vi "as_saveStimList.vi"(4 "error in (no error)":errorcluster, 6 "Stimulus List":dbl[][](array[numeric]), 7 "Path In":path) -> (0 "error out":errorcluster, 3 "Path":path)   [LabVIEW 2009]
uses:
  <vilib>/Utility/file.llb/Write To Spreadsheet File (DBL).vi
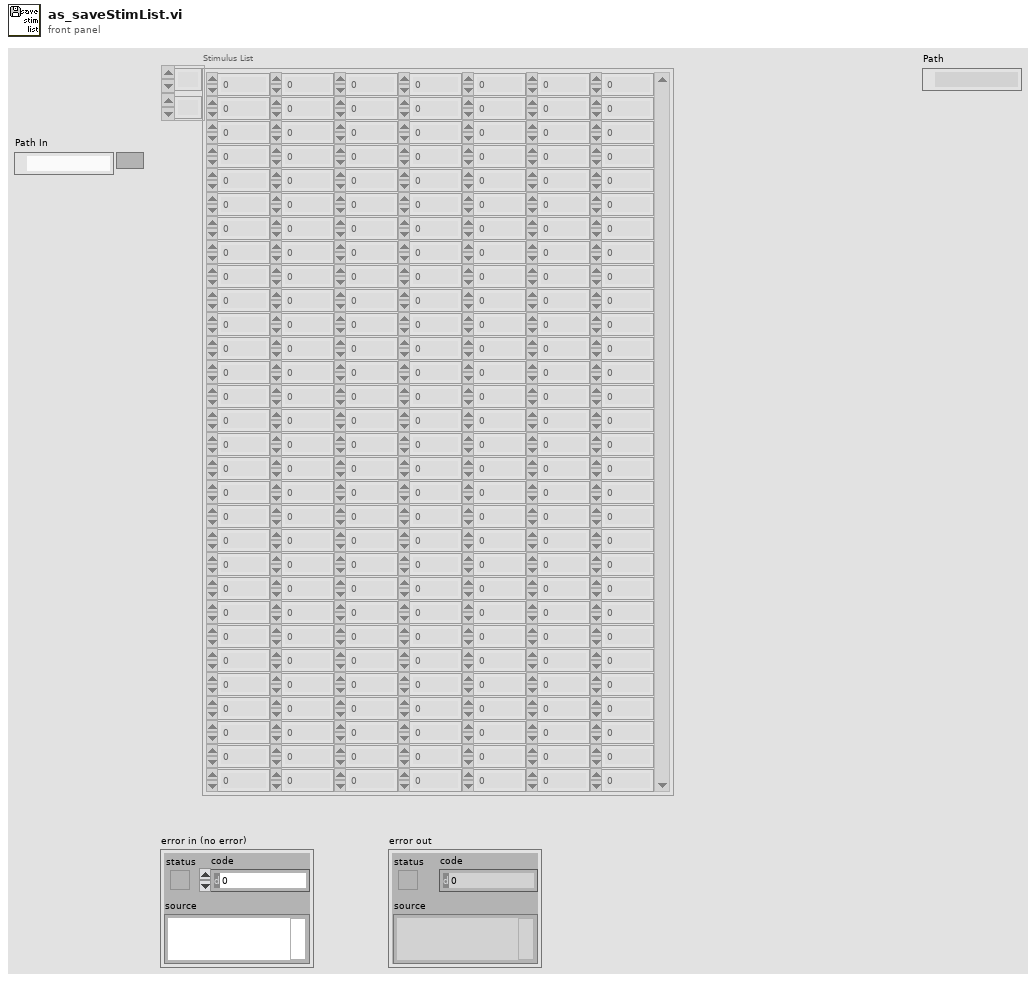
[diagram p1: front panel]
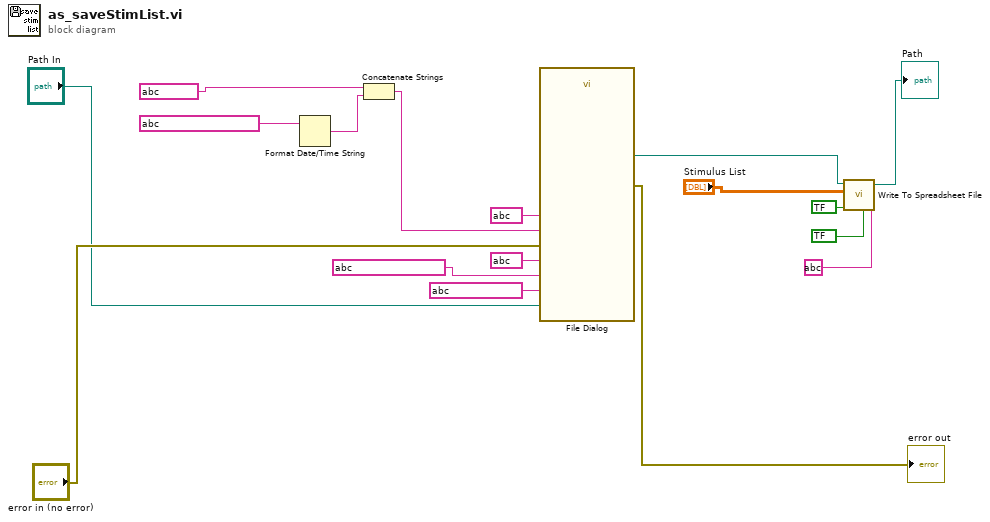
[diagram p0: block diagram]
diagram:
  n1 = Format Date/Time String(time format string (%c)=string ?) -> (date/time string=w12:string)  [unwired: 2 in]
  n2 = Concatenate Strings(string ?, w12) -> (w11:string)
  n3 = call "File Dialog"("start path"="Path In", "prompt"=string ?, "button label"=string ?, "default name"=w11, "error in"="error in (no error)", "pattern (all files)"=string ?, "pattern label"=string ?) -> ("selected path"=w7:path, "error out"=→"error out":errorcluster)  [unwired: 5 in, 2 out]
  n4 = call-poly <vilib>:"Write To Spreadsheet File.vi"("delimiter (\\t)"=string ? ("delimiter (\\t)"), "transpose? (no:F)"=bool ?, "append to file? (new file:F)"=bool ?, "2D data"="Stimulus List", "file path (dialog if empty)"=w7) -> ("new file path (Not A Path if cancelled)"=→"Path":path)  [unwired: 3 in]
